vi "Cast Data Class.vi"(8 "error in":errorcluster, 10 "Type":string, 11 "Alicat Device in":refnum<class "Alicat Device.lvclass">) -> (0 "error out":errorcluster, 2 "Alicat Data Out":refnum<class "Alicat Data.lvclass">, 3 "Alicat Device out":refnum<class "Alicat Device.lvclass">)   [LabVIEW 2015, in "Alicat Device.lvclass"]
doc: "Load the data class dynamically. If the class can not be found, load the default class (Alicat Data) so everything does not break."
uses:
  Alicat Device.lvclass
  Data/Alicat Data.lvclass
  Alicat Device.lvclass/Alicat Device.ctl
  Data/M/M data.lvclass
  Data/P/P.lvclass
  Data/P/P.lvclass/P.ctl
  Data/Alicat Data.lvclass/Alicat Data.ctl
  Data/P/Write convertPtoQ.vi
  Data/P/Write formula.vi
  Data/Accessors/Write ID.vi
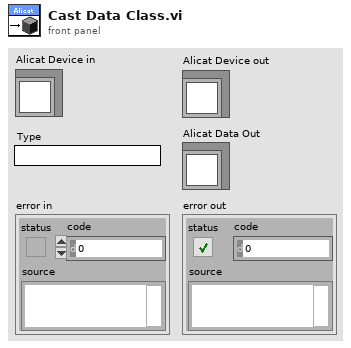
[diagram p1: front panel]
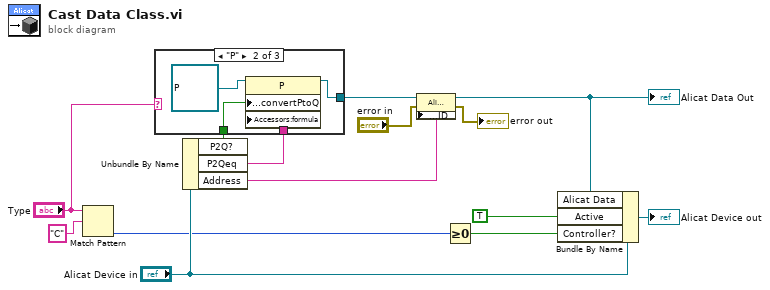
[diagram p0: block diagram]
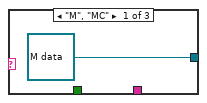
[diagram p2: hidden frame]
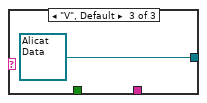
[diagram p3: hidden frame]
diagram:
  n1 = Match Pattern(string="Type", regular expression="C") -> (offset past match=w8:i32)  [unwired: 1 in, 3 out]
  n2 = Unbundle By Name("Alicat Device in") -> ("P2Q?"=w2:bool, "P2Qeq"=w1:string, "Address"=w11:string)
  n3 = case shown="\"P\"" "Type" {
    tunnel: [refnum<class "M data.lvclass"> refnum ("M Data") w16 refnum<class "Alicat Data.lvclass"> refnum ("Alicat Data")] -> w13
    tunnel: w2 -> [_ w18 _]
    tunnel: w1 -> [_ w17 _]
    frame "M", "MC" {
    }
    frame "P" {
      n4 = property class="P"(reference=refnum<class "P.lvclass"> refnum ("P.lvclass"), "Accessors:convertPtoQ"=w18, "Accessors:formula"=w17) -> (reference out=w16:refnum<class "P.lvclass">)  [unwired: 1 in, 1 out]
    }
    frame "V", Default {
    }
  }
  n5 = property class="Alicat Data"(reference=w13, error in="error in", "Accessors:ID"=w11) -> (reference out=w10:refnum<class "Alicat Data.lvclass">, error out=→"error out":errorcluster)
  "Alicat Data Out" <- w10
  n6 = Greater Or Equal To 0?(x=w8) -> (x >= 0?=w6:bool)
  n7 = Bundle By Name(cluster="Alicat Device in", "Alicat Data"=w10, "Active"=TRUE, "Controller?"=w6) -> (→"Alicat Device out":refnum<class "Alicat Device.lvclass">)
